vi "Course Adjust.vi"(9 "Within X Degrees":dbl, 10 "Yaw prop feedback":dbl=0.005, 11 "Drive Metrics In":T1) -> (3 "Drive Train Metrics Out":T1)   [LabVIEW 2014]
uses:
  Drive Train Metrics.ctl
  CmdFlag.ctl
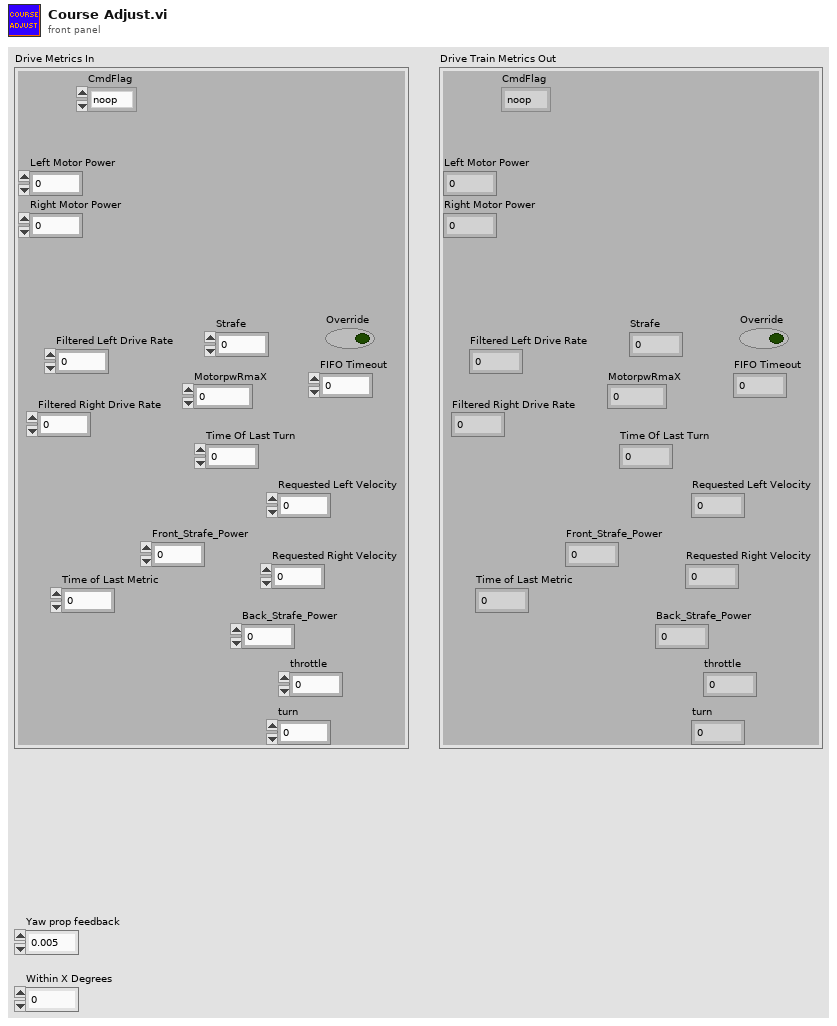
[diagram p1: front panel]
types:
  T1 = typedef "Drive Train Metrics.ctl" = cluster{"CmdFlag":T2, "Right Motor Power":dbl, "Left Motor Power":dbl, "Filtered Left Drive Rate":dbl, "Filtered Right Drive Rate":dbl, "Time of Last Metric":u32, "FIFO Timeout":i32, "Requested Left Velocity":dbl, "Requested Right Velocity":dbl, "throttle":dbl, "turn":dbl, "MotorpwRmaX":i32, "Strafe":dbl, "Override":bool, "Time Of Last Turn":dbl, "Front_Strafe_Power":dbl, "Back_Strafe_Power":dbl}
  T2 = typedef "CmdFlag.ctl" = enum16{"noop", "suspend", "resume"}
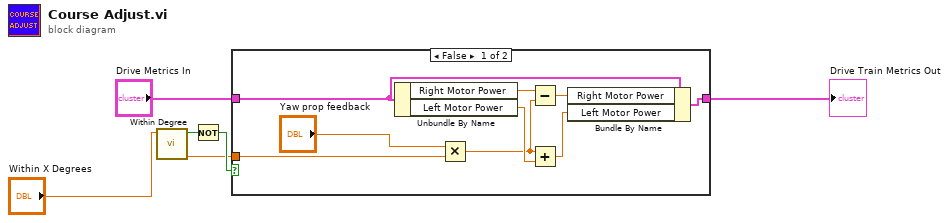
[diagram p0: block diagram]
diagram:
  n1 = call "Within Degree.vi"("Within X Degrees"="Within X Degrees") -> ("Yaw"=w3:dbl, "Boolean"=w4:bool)  [unwired: 9 in]
  n2 = Not(x=w4) -> (.not. x?=w5:bool)
  n3 = case shown="False" w5 {
    tunnel: "Drive Metrics In" -> [w10 w16]
    tunnel: [w9 w16] -> w1
    tunnel: w3 -> [w14 _]
    frame False {
      n4 = Unbundle By Name(w10) -> ("Right Motor Power"=w11:dbl, "Left Motor Power"=w13:dbl)
      n5 = Multiply(x="Yaw prop feedback", y=w14) -> (x*y=w12:dbl)
      n6 = Subtract(x=w11, y=w12) -> (x-y=w8:dbl)
      n7 = Add(x=w12, y=w13) -> (x+y=w7:dbl)
      n8 = Bundle By Name(cluster=w10, "Right Motor Power"=w8, "Left Motor Power"=w7) -> (w9:T1)
    }
    frame True {
    }
  }
  "Drive Train Metrics Out" <- w1
